vi "Set Waveform Vertical Offset.vi"(8 "error in (no error)":errorcluster, 9 "Offset Divisions":dbl, 10 "Analog Channels":T1, 11 "DPO4104 in":refnum<class "DPO4104.lvclass">) -> (0 "error out":errorcluster, 3 "DPO4104 out":refnum<class "DPO4104.lvclass">)   [LabVIEW 2018, in "DPO4104.lvlib" / "DPO4104.lvclass"]
doc: "This Override is used to change the vertical placement individual waveforms."
uses:
  DPO4104.lvclass
  PPLs/Oscilloscope/Parent/Oscilloscope.lvlibp/Custom Controls/Analog Channels.ctl
  PPLs/Oscilloscope/Parent/Oscilloscope.lvlibp/Oscilloscope.lvclass
  <instrlib>/Tektronix DPO MSO 2000 4000 Series/Tektronix DPO MSO 2000 4000 Series.lvlib
  C:/Projects/LabVIEW/PPLs/Oscilloscope/Parent/Oscilloscope.lvlibp/Oscilloscope.lvclass
  PPLs/Oscilloscope/Parent/Oscilloscope.lvlibp
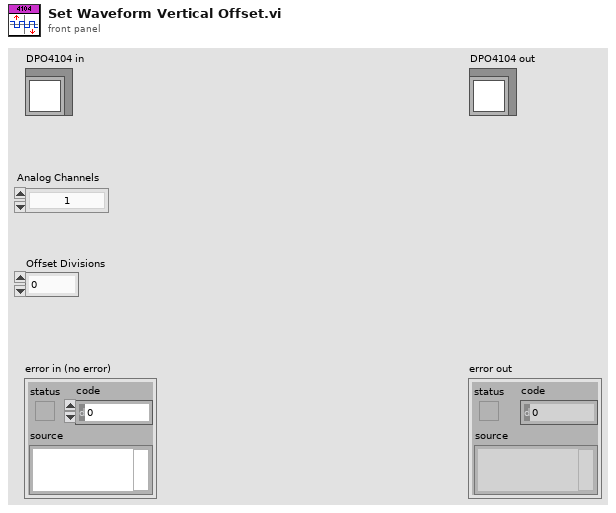
[diagram p1: front panel]
types:
  T1 = typedef "Oscilloscope.lvlibp/Analog Channels.ctl" = enum16{"1", "2", "3", "4", "5", "6", "7", "8", "9", "10", "11", "12", "13", "14", "15", "16"}
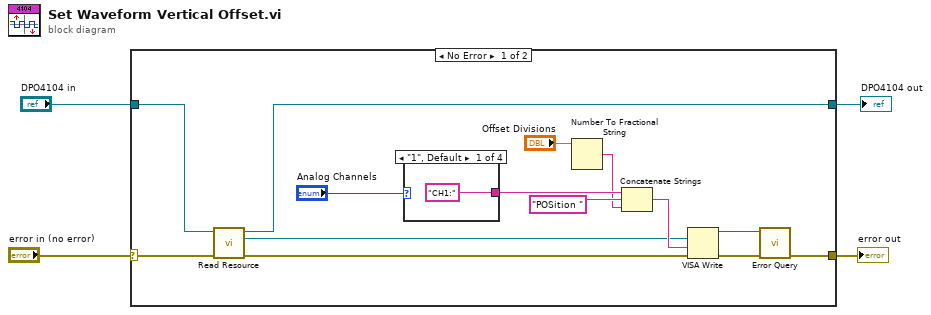
[diagram p0: block diagram]
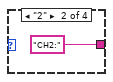
[diagram p2: hidden frame]
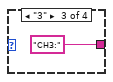
[diagram p3: hidden frame]
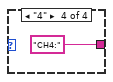
[diagram p4: hidden frame]
diagram:
  n1 = case shown="No Error" "error in (no error)" {
    selector: "error in (no error)" -> [w18 w24]
    tunnel: [w6 w24] -> w3
    tunnel: [w16 w23] -> w2
    tunnel: "DPO4104 in" -> [w17 w23]
    frame No Error {
      n2 = call "Read Resource.vi"("error in (no error)"=w18, "Oscilloscope in"=w17) -> ("error out"=w7:errorcluster, "Resource"=w5:refnum<visa-resource-name>, "Oscilloscope out"=w16:refnum<class "DPO4104.lvclass">)  [unwired: 7 in]
      n3 = case shown="\"1\", Default" "Analog Channels" {
        tunnel: ["CH1:" "CH2:" "CH3:" "CH4:"] -> w10
        frame "1", Default {
        }
        frame "2" {
        }
        frame "3" {
        }
        frame "4" {
        }
      }
      n4 = Number To Fractional String(number="Offset Divisions") -> (F-format string=w8:string)  [unwired: 3 in]
      n5 = Concatenate Strings(w10, "POSition " ("string"), w8) -> (w11:string)
      n6 = VISA Write(VISA resource name=w5, write buffer=w11, error in (no error)=w7) -> (VISA resource name out=w13:refnum<visa-resource-name>, error out=w12:errorcluster)  [unwired: 1 out]
      n7 = call <instrlib>:"Error Query.vi"("error in (no error)"=w12, "VISA resource name"=w13) -> ("error out"=w6:errorcluster)  [unwired: 6 in, 3 out]
    }
    frame Error {
    }
  }
  "error out" <- w3
  "DPO4104 out" <- w2
